vi "Description Image Source.vi"(8 "Error In":errorcluster, 11 "File Stem":string) -> (0 "Error Out":errorcluster, 3 "Description Image Src":string)   [LabVIEW 2018, in "Scripts.lvlib"]
uses:
  Scripts.lvlib
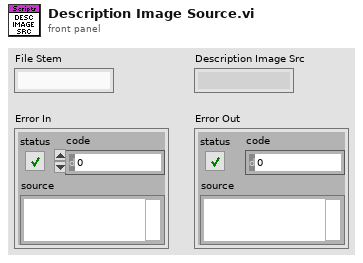
[diagram p1: front panel]
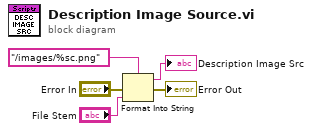
[diagram p0: block diagram]
diagram:
  n1 = Format Into String(format string="/images/%sc.png", error in="Error In", "File Stem") -> (resulting string=→"Description Image Src":string, error out=→"Error Out":errorcluster)  [unwired: 1 in]
